vi "Scalar Data to String.vi"(11 "Data":variant) -> (0 "error out":errorcluster, 2 "Value String":string)   [LabVIEW 2019, in "VariantExtensions.lvlib"]
doc: "<License>\nCopyright © 2017 Composed Systems, LLC | All rights reserved\nwww.composed.io\n\nAuthor: Ethan Stern <ethan.stern@composed.io>\n\nThis software is provided \"AS IS\" WITHOUT WARRANTIES, either express or implied, AND IS FOR EDUCATIONAL PURPOSES ONLY.\n</License>"
uses:
  <vilib>/gpm_packages/@cs/variant/Source/VariantExtensions.lvlib
  <vilib>/Utility/Data Type/NI_Data Type.lvlib
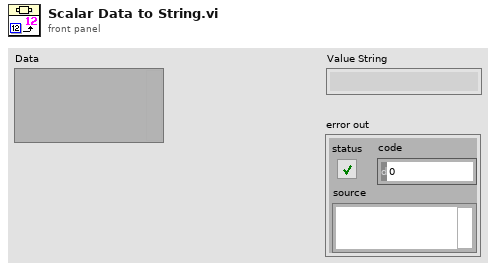
[diagram p1: front panel]
types:
  T1 = typedef "NI_Data Type.lvlib/Data Type.ctl" = enum8{"Invalid Type", "Void", "I8", "I16", "I32", "I64", "U8", "U16", "U32", "U64", "Single Float", "Double Float", "Extended Float", "Single Complex", "Double Complex", "Extended Complex", "Enum U8", "Enum U16", "Enum U32", "Enum U64", "Single Float With Unit", "Double Float With Unit", "Extended Float With Unit", "Single Complex with Unit", "Double Complex with Unit", "Extended Complex with Unit", "Boolean", "String", "Path", "Picture", "Tag", "Array", "Cluster", "Variant", "LV Variant", "Waveform", "Timestamp", "Digital Waveform", "Digital Data", "ExpressData", "Refnum", "External Data", "VI", "Poly VI", "LabVIEW Class Instance", "Fixed Point", "Set Collection", "Map Collection"}
  T2 = typedef "NI_Data Type.lvlib/Refnum Type.ctl" = enum16{"NotARefnum", "UnknownRefnum", "Generic", "Datalog", "ByteStream", "Device", "Occurence", "TCPNetConnection", "Auto", "Menu", "Imaq", "Hardware", "DataSocket", "Visa", "IVI", "UDPNetConnection", "Notifier", "Queue", "Irda", "EventReg", "DotNet", "UserEvent", "Callback", "UNUSED_EMPTY_POSITION", "BlueToothNetConnection", "LVObjApp", "LVObjVI", "LVObjUnknown", "GenericClass", "UserDefinedRefnumTag", "DataValue", "RT FIFO", "TDMS File", "PythonSessionRefnum"}
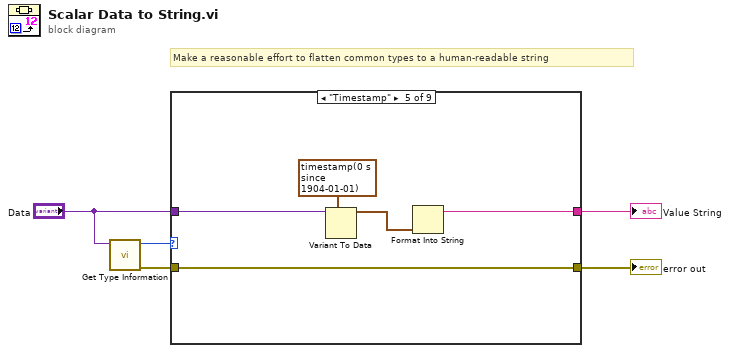
[diagram p0: block diagram]
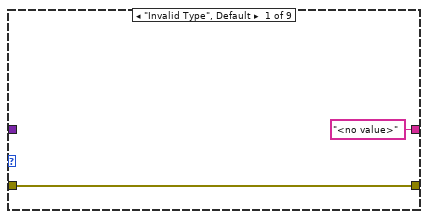
[diagram p2: hidden frame]
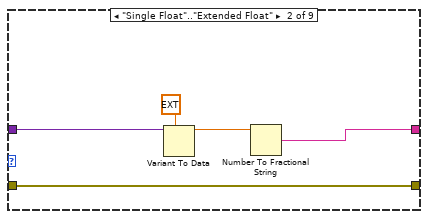
[diagram p3: hidden frame]
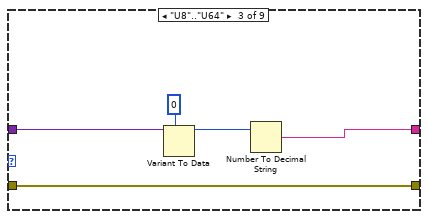
[diagram p4: hidden frame]
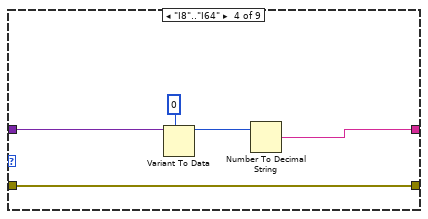
[diagram p5: hidden frame]
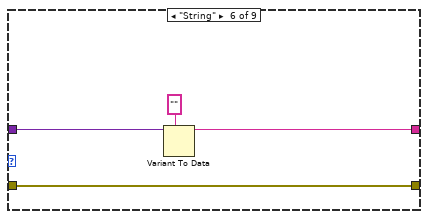
[diagram p6: hidden frame]
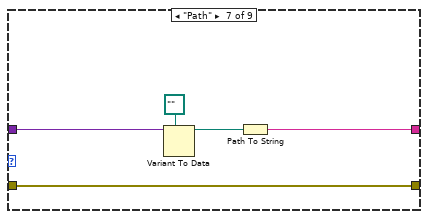
[diagram p7: hidden frame]
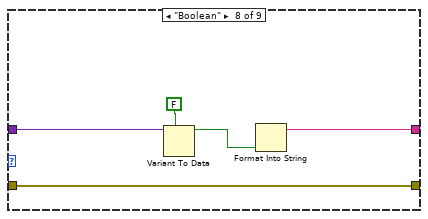
[diagram p8: hidden frame]
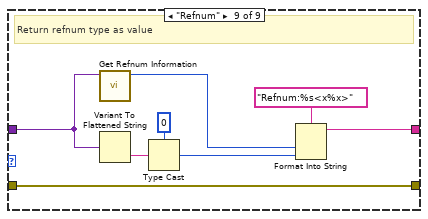
[diagram p9: hidden frame]
diagram:
  # "Make a reasonable effort to flatten common types to a human-readable string"
  n1 = call <vilib>:"Get Type Information.vi"("variant"="Data") -> ("error out"=w3:errorcluster, "type"=w2:T1)  [unwired: 6 in, 3 out]
  n2 = case shown="\"Timestamp\"" w2 {
    tunnel: "Data" -> [_ w11 w16 w21 w26 w30 w35 w40 w45]
    tunnel: ["<no value>" w10 w15 w20 w23 w29 w33 w37 w47] -> w4
    tunnel: w3 -> [w7 w8 w13 w18 w25 w28 w32 w39 w49]
    tunnel: [w7 w8 w13 w18 w25 w28 w32 w39 w49] -> w1
    frame "Invalid Type", Default {
    }
    frame "Single Float".."Extended Float" {
      n3 = Variant To Data(type=ext 0.0, Variant=w11) -> (data=w9:ext)  [unwired: 1 in, 1 out]
      n4 = Number To Fractional String(number=w9) -> (F-format string=w10:string)  [unwired: 3 in]
    }
    frame "U8".."U64" {
      n5 = Variant To Data(type=u64 0, Variant=w16) -> (data=w14:u64)  [unwired: 1 in, 1 out]
      n6 = Number To Decimal String(number=w14) -> (decimal integer string=w15:string)  [unwired: 1 in]
    }
    frame "I8".."I64" {
      n7 = Variant To Data(type=i64 0, Variant=w21) -> (data=w19:i64)  [unwired: 1 in, 1 out]
      n8 = Number To Decimal String(number=w19) -> (decimal integer string=w20:string)  [unwired: 1 in]
    }
    frame "Timestamp" {
      n9 = Variant To Data(type=timestamp(0 s since 1904-01-01), Variant=w26) -> (data=w24:timestamp)  [unwired: 1 in, 1 out]
      n10 = Format Into String(w24) -> (resulting string=w23:string)  [unwired: 3 in, 1 out]
    }
    frame "String" {
      n11 = Variant To Data(type="", Variant=w30) -> (data=w29:string)  [unwired: 1 in, 1 out]
    }
    frame "Path" {
      n12 = Variant To Data(type=path "", Variant=w35) -> (data=w34:path)  [unwired: 1 in, 1 out]
      n13 = Path To String(path=w34) -> (string=w33:string)
    }
    frame "Boolean" {
      n14 = Variant To Data(type=FALSE, Variant=w40) -> (data=w38:bool)  [unwired: 1 in, 1 out]
      n15 = Format Into String(w38) -> (resulting string=w37:string)  [unwired: 3 in, 1 out]
    }
    frame "Refnum" {
      # "Return refnum type as value"
      n16 = call <vilib>:"Get Refnum Information.vi"("variant"=w45) -> ("reference type"=w48:T2)  [unwired: 7 in, 3 out]
      n17 = Variant To Flattened String(Variant=w45) -> (data string=w44:string)  [unwired: 1 out]
      n18 = Type Cast(type=u32 0, x=w44) -> (*(type *) &x=w42:u32)
      n19 = Format Into String(format string="Refnum:%s<x%x>", w48, w42) -> (resulting string=w47:string)  [unwired: 2 in, 1 out]
    }
  }
  "error out" <- w1
  "Value String" <- w4
